vi "SingleChannel PI Controller.vi"(9 "Integral Coefficient a[k]":fxp<+/-,18,2>, 10 "Integral Coefficient b[k]":fxp<+/-,18,1>, 11 "input data":fxp<+/-,21,6>) -> (3 "output data":fxp<+/-,20,5> format="%.31g")   [LabVIEW 2011, in "Filter VIs.lvlib"]
doc: "----------------------\n\nThis filter is configured as follows:\n\n<b>Filter Configuration</b>\nType: Single Rate\nStructure: IIR Cascaded Second-Order Sections Form II Transposed\n\n<b>Input Data Type</b>\nType: fixed-point <±,20,5> [-1.600000E+1,1.599997E+1]:3.051758E-5\n\n<b>Output Data Type</b>\nType: fixed-point <±,20,5> [-1.600000E+1,1.599997E+1]:3.051758E-5\nRounding mode: Round-Half-Even\nOverflow mode: Wrap\n\n<b>Implementation</b>\nNumber of channels: 1\nMaximum input sampling rate per channel @ 40MHz: 8MHz\nGain processing: On Target\nMethod: Multiply-Accumulate\n\n<b>Execution Mode</b>\nOutside single-cycle Timed Loop\nThroughput: 5 cycles/call\n\n<b>Estimated Resources</b>\n2 24x32 multiplier"
uses:
  Filter VIs.lvlib
  <vilib>/Platform/TimedLoop/XDataNode/timing_clust.ctl
  <vilib>/Platform/TimedLoop/XDataNode/nitl_modes.ctl
  <vilib>/Platform/TimedLoop/XDataNode/wakeup.ctl
  <vilib>/Platform/TimedLoop/XDataNode/XDataNode.xnode
  <vilib>/Platform/TimedLoop/XDataNode/XDNodeRunTimeDep.lvlib
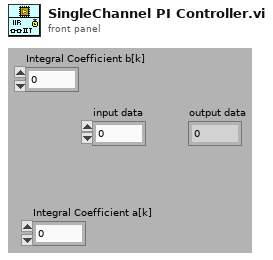
[diagram p1: front panel]
types:
  T1 = typedef "XDNodeRunTimeDep.lvlib/timing_clust.ctl" = cluster{"Expected End [f-1]":u64, "Actual End [f-1]":u64, "Finished Late? [f-1]":bool, "Expected End [i-1]":u64, "Actual End [i-1]":u64, "Finished Late? [i-1]":bool, "Expected Start [i]":u64, "Actual Start [i]":u64, "Expected Start [f]":u64, "Actual Start [f]":u64, "Source Name":string, "Structure Name":string, "Period":i64, "Deadline":i64, "Offset":i64, "Start":i64, "Priority":i32, "Timeout":i32, "Mode":T2, "Wakeup Reason":T3, "Error":errorcluster, "Source Type":string, "Secondary Source Type":string, "Global End Time":u64, "Global Start Time":u64, "Frame Duration":u64, "Iteration Duration":u64, "Assigned CPU":i32, "I/O Scan Engine Mode":u32}
  T2 = typedef "XDNodeRunTimeDep.lvlib/nitl_modes.ctl" = enum32{"No Change", "Process missed periods, maintain original phase", "Discard missed periods, maintain original phase", "Process missed periods, ignore original phase", "Discard missed periods, ignore original phase"}
  T3 = typedef "XDNodeRunTimeDep.lvlib/wakeup.ctl" = enum32{"Normal", "Aborted", "Asynchronous wakeup", "Timing source error", "Timed loop error", "Timeout"}
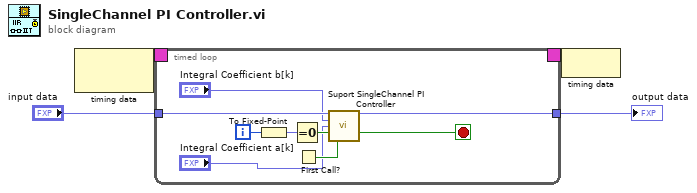
[diagram p0: block diagram]
diagram:
  n1 = node-c288() -> (w2:T1)  [unwired: 1 in]
  n2 = timed-loop "SCTL" {
    tunnel: "input data" -> [w8]
    tunnel: [w7] -> w3
    timing: w2 -> [_]
    timing-out: [_] -> w1
    i -> [w13]
    stop <- w9 stop-if-true
    n3 = To Fixed-Point(number=w13) -> (fixed-point=w12:fxp<+,12,12>)  [unwired: 1 out]
    n4 = Equal To 0?(x=w12) -> (x = 0?=w11:bool)
    n5 = First Call?() -> (First Call?: T/F=w10:bool)
    n6 = call "Suport SingleChannel PI Controller.vi"("input data"=w8, "Integral Coefficient b[k]"="Integral Coefficient b[k]", "Integral Coefficient a[k]"="Integral Coefficient a[k]", "input valid"=w11, "reset"=w10) -> ("output data"=w7:fxp<+/-,20,5>, "output valid"=w9:bool)  [unwired: 8 in, 1 out]
  }
  "output data" <- w3
  n7 = node-c288(w1) -> ()
